vi "Create Archiving Transaction List.vi"(8 "Volts Only":bool, 9 "Combined LBCBs":bool, 10 "Hold":T2, 11 "Number of LBCBs":T1) -> (2 "Transactions":T3[](array[typedef]))   [LabVIEW 2009]
uses:
  Dataset Transaction Id.ctl
  Dataset Source.ctl
  Dataset Type.ctl
  Apps/Yes No Button.ctl
  Data Access Objects/Application/Number Of LBCBs.ctl
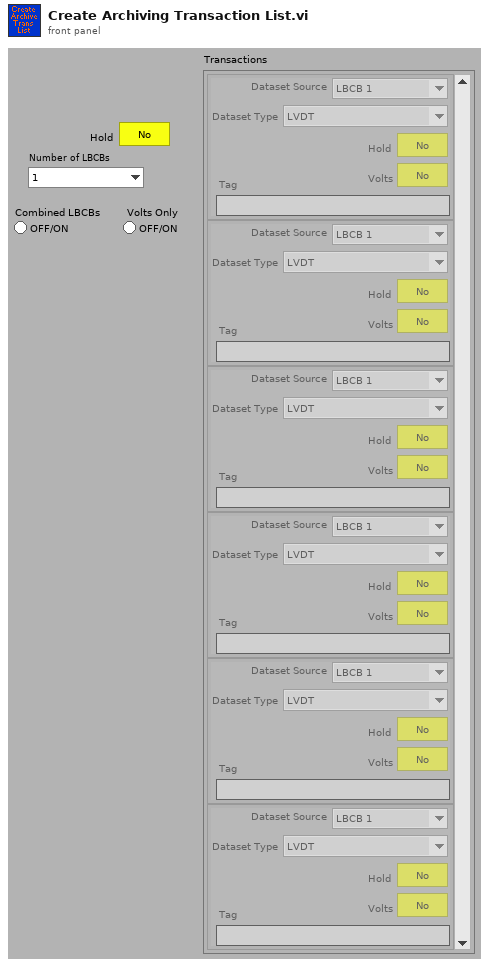
[diagram p1: front panel]
types:
  T1 = typedef "Number Of LBCBs.ctl" = enum16{"1", "2"}
  T2 = typedef "Yes No Button.ctl" = bool
  T3 = typedef "Dataset Transaction Id.ctl" = cluster{"Dataset Source":T4, "Dataset Type":T5, "Hold":T2, "Volts":T2, "Tag":string}
  T4 = typedef "Dataset Source.ctl" = enum16{"LBCB 1", "LBCB 2", "Combined", "External Sensors"}
  T5 = typedef "Dataset Type.ctl" = enum16{"LVDT", "Load Cell", "Actuator Command", "Servo Error", "Displacement Command", "Displacement", "Force"}
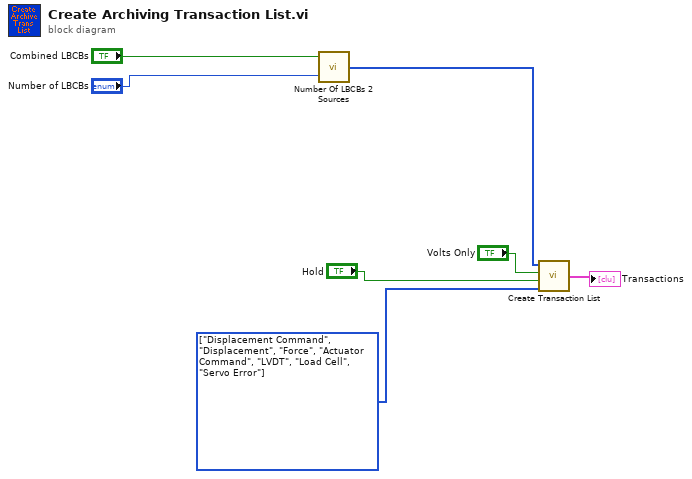
[diagram p0: block diagram]
diagram:
  w5 = T5[] [enum."Displacement Command", enum."Displacement", enum."Force", enum."Actuator Command", enum."LVDT", enum."Load Cell", enum."Servo Error"] items=["LVDT", "Load Cell", "Actuator Command", "Servo Error", "Displacement Command", "Displacement", "Force"] ("Types")
  n1 = call "Number Of LBCBs 2 Sources.vi"("Number of LBCBs"="Number of LBCBs", "Combined LBCBs"="Combined LBCBs") -> ("Sources"=w6:T4[])
  n2 = call "Create Transaction List.vi"("Types"=w5, "Hold"="Hold", "Volts"="Volts Only", "Sources"=w6) -> ("Transactions"=→"Transactions":T3[])
